vi "High 4 Bits Write.vi"(6 "E?E1:E2 (E1)":bool=TRUE, 9 "RS":bool, 10 "LCD data/cmd":u8 format="%.0x", 11 "device connection map":T1={"RS"="RS", "R/W"="RW", "E1"="E1", "E2"="E2", "DB4"="DB4", "DB5"="DB5", "DB6"="DB6", "DB7"="DB7"}) -> ()   [LabVIEW 2017, in "HD44780 FPGA.lvlib"]
uses:
  HD44780 FPGA.lvlib
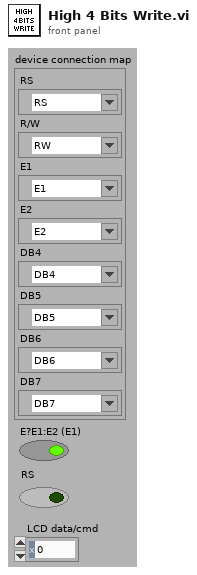
[diagram p1: front panel]
types:
  T1 = cluster{"RS":refnum<k21>, "R/W":refnum<k21>, "E1":refnum<k21>, "E2":refnum<k21>, "DB4":refnum<k21>, "DB5":refnum<k21>, "DB6":refnum<k21>, "DB7":refnum<k21>}
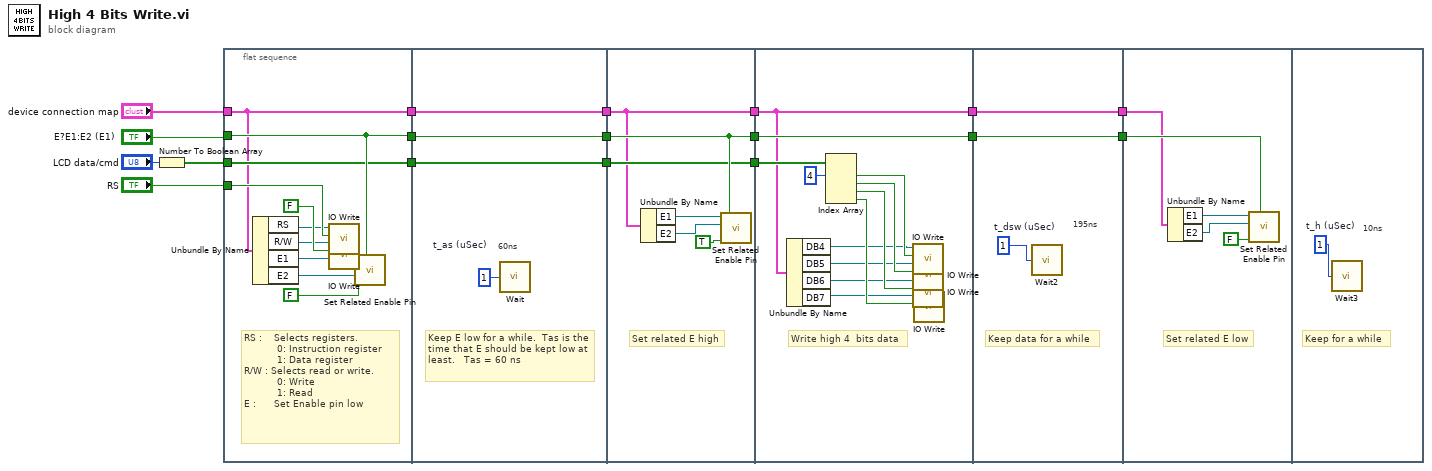
[diagram p0: block diagram]
diagram:
  n1 = Number To Boolean Array(number="LCD data/cmd") -> (Boolean array=w17:bool[])
  n2 = flat-sequence {
    tunnel: [w24] -> w14
    tunnel: [w25] -> w13
    tunnel: [w19] -> w4
    tunnel: w17 -> [w24]
    tunnel: "RS" -> [w28]
    tunnel: "E?E1:E2 (E1)" -> [w25]
    tunnel: "device connection map" -> [w19]
    tunnel: w14 -> [w31]
    tunnel: [w31] -> w12
    tunnel: w13 -> [w30]
    tunnel: [w30] -> w11
    tunnel: [w29] -> w5
    tunnel: w4 -> [w29]
    tunnel: w12 -> [w36]
    tunnel: [w36] -> w10
    tunnel: w11 -> [w37]
    tunnel: [w37] -> w9
    tunnel: [w35] -> w6
    tunnel: w5 -> [w35]
    tunnel: w10 -> [w49]
    tunnel: w9 -> [w44]
    tunnel: [w44] -> w8
    tunnel: w6 -> [w43]
    tunnel: [w43] -> w2
    tunnel: w8 -> [w52]
    tunnel: [w52] -> w7
    tunnel: [w51] -> w3
    tunnel: w2 -> [w51]
    tunnel: w7 -> [w58]
    tunnel: w3 -> [w54]
    frame #0 {
      # "RS :    Selects registers.\n           0: Instruction register  \n           1: Data register\nR/W : Selects read or write.\n           0: Write\n           1: Read\nE :      Set Enable pin low"
      n3 = Unbundle By Name(w19) -> ("RS"=w23:refnum<k21>, "R/W"=w22:refnum<k21>, "E1"=w21:refnum<k21>, "E2"=w20:refnum<k21>)
      n4 = call "IO Write.vi"("data"=w28, "I/O"=w23) -> ()  [unwired: 10 in]
      n5 = call "IO Write.vi"("data"=FALSE, "I/O"=w22) -> ()  [unwired: 10 in]
      n6 = call "Set Related Enable Pin.vi"("E?E1:E2"=w25, "data"=FALSE, "E2"=w20, "E1"=w21) -> ()  [unwired: 8 in]
    }
    frame #1 {
      w32 = u32 1  # t_as (uSec)
      # "60ns"
      # "Keep E low for a while.  Tas is the time that E should be kept low at least.   Tas = 60 ns"
      n7 = call "Wait"("Count(uSec)"=w32) -> ()  [unwired: 1 out]
    }
    frame #2 {
      # "Set related E high"
      n8 = Unbundle By Name(w35) -> ("E1"=w34:refnum<k21>, "E2"=w33:refnum<k21>)
      n9 = call "Set Related Enable Pin.vi"("E?E1:E2"=w37, "data"=TRUE, "E2"=w33, "E1"=w34) -> ()  [unwired: 8 in]
    }
    frame #3 {
      # "Write high 4  bits data"
      n10 = Unbundle By Name(w43) -> ("DB4"=w42:refnum<k21>, "DB5"=w41:refnum<k21>, "DB6"=w40:refnum<k21>, "DB7"=w39:refnum<k21>)
      n11 = Index Array(array=w49, index #1=4 ("index")) -> (element #1=w48:bool, element #2=w47:bool, element #3=w46:bool, element #4=w45:bool)  [unwired: 3 in]
      n12 = call "IO Write.vi"("data"=w48, "I/O"=w42) -> ()  [unwired: 10 in]
      n13 = call "IO Write.vi"("data"=w47, "I/O"=w41) -> ()  [unwired: 10 in]
      n14 = call "IO Write.vi"("data"=w46, "I/O"=w40) -> ()  [unwired: 10 in]
      n15 = call "IO Write.vi"("data"=w45, "I/O"=w39) -> ()  [unwired: 10 in]
    }
    frame #4 {
      w53 = u32 1  # t_dsw (uSec)
      # "Keep data for a while"
      # "195ns"
      n16 = call "Wait2"("Count(uSec)"=w53) -> ()  [unwired: 1 out]
    }
    frame #5 {
      # "Set related E low"
      n17 = Unbundle By Name(w54) -> ("E1"=w56:refnum<k21>, "E2"=w55:refnum<k21>)
      n18 = call "Set Related Enable Pin.vi"("E?E1:E2"=w58, "data"=FALSE, "E2"=w55, "E1"=w56) -> ()  [unwired: 8 in]
    }
    frame #6 {
      w59 = u32 1  # t_h (uSec)
      # "Keep for a while"
      # "10ns"
      n19 = call "Wait3"("Count(uSec)"=w59) -> ()  [unwired: 1 out]
    }
  }
